vi "Extract Rows.vi"(8 "String":string[](array[string]), 9 "Saving":bool[](array[boolean]), 10 "Enum":enum16{"0-6", "6-6", "6-12", "6-18"}(ring), 11 "Board Index":dbl[](array[numeric])) -> (0 "String Output":string[](array[string]), 2 "Boolean Array":bool[](array[boolean]), 3 "Array":dbl[](array[numeric]))   [LabVIEW 2012]
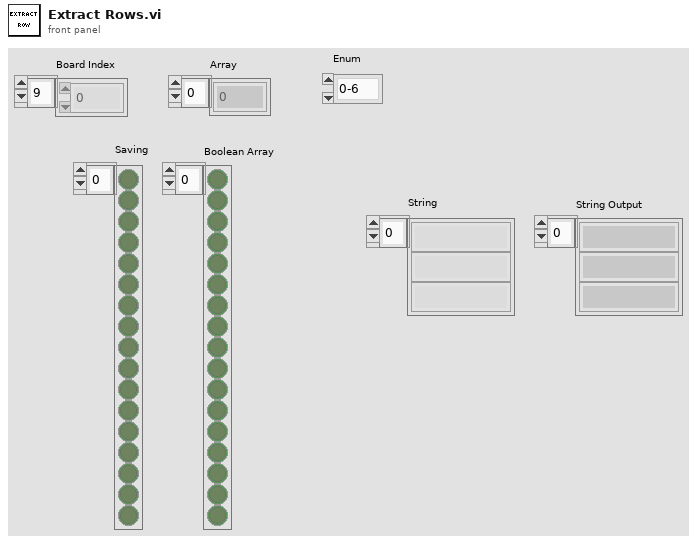
[diagram p1: front panel]
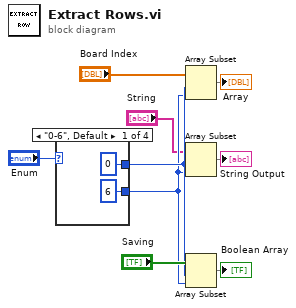
[diagram p0: block diagram]
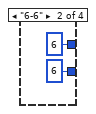
[diagram p2: hidden frame]
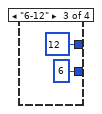
[diagram p3: hidden frame]
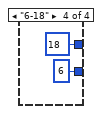
[diagram p4: hidden frame]
diagram:
  n1 = case shown="\"0-6\", Default" "Enum" {
    tunnel: [0 6 12 18] -> w4
    tunnel: [6 6 6 6] -> w3
    frame "0-6", Default {
    }
    frame "6-6" {
    }
    frame "6-12" {
    }
    frame "6-18" {
    }
  }
  n2 = Array Subset(array="Board Index", index=w4, length=w3) -> (→"Array":dbl[])
  n3 = Array Subset(array="String", index=w4, length=w3) -> (→"String Output":string[])
  n4 = Array Subset(array="Saving", index=w4, length=w3) -> (→"Boolean Array":bool[])
